vi "Conversao Ms to Hora texto.vi"(1 "TRUE=HORA\nFALSE=GRAU":bool, 2 "PrecDEC":dbl caption="DEC arcsec" format="%.3g") -> (0 "Hora/Graus Texto Decimal":string)   [LabVIEW 2018]
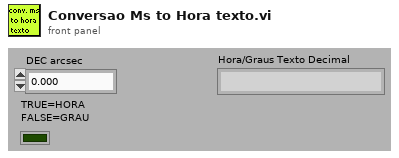
[diagram p1: front panel]
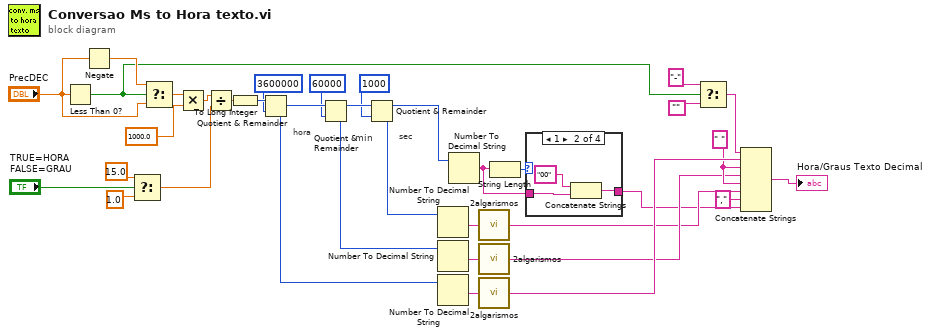
[diagram p0: block diagram]
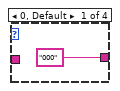
[diagram p2: hidden frame]
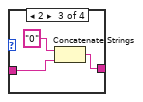
[diagram p3: hidden frame]
diagram:
  w22 = " " ("string")
  # "sec"
  # "min"
  # "hora"
  n1 = Less Than 0?(x="PrecDEC") -> (x < 0?=w9:bool)
  n2 = Negate(x="PrecDEC") -> (-x=w11:dbl)
  n3 = Select(t=15.0 ("y"), s="TRUE=HORA\nFALSE=GRAU", f=1.0 ("y")) -> (s? t:f=w1:dbl)
  n4 = Select(t=w11, s=w9, f="PrecDEC") -> (s? t:f=w13:dbl)
  n5 = Multiply(x=w13, y=1000.0) -> (x*y=w6:dbl)
  n6 = Divide(x=w6, y=w1) -> (x/y=w5:dbl)
  n7 = To Long Integer(number=w5) -> (32bit integer=w35:i32)
  n8 = Quotient & Remainder(x=w35, y=3600000) -> (x-y*floor(x/y)=w33:i32, floor(x/y)=w29:i32)
  n9 = Quotient & Remainder(x=w33, y=60000) -> (x-y*floor(x/y)=w31:i32, floor(x/y)=w25:i32)
  n10 = Quotient & Remainder(x=w31, y=1000) -> (x-y*floor(x/y)=w18:i32, floor(x/y)=w24:i32)
  n11 = Number To Decimal String(number=w24) -> (decimal integer string=w26:string)  [unwired: 1 in]
  n12 = Number To Decimal String(number=w25) -> (decimal integer string=w27:string)  [unwired: 1 in]
  n13 = Number To Decimal String(number=w29) -> (decimal integer string=w28:string)  [unwired: 1 in]
  n14 = Number To Decimal String(number=w18) -> (decimal integer string=w16:string)  [unwired: 1 in]
  n15 = call "2algarismos.vi"("entrada"=w26) -> ("saida"=w20:string)
  n16 = call "2algarismos.vi"("entrada"=w27) -> ("saida"=w21:string)
  n17 = call "2algarismos.vi"("entrada"=w28) -> ("saida"=w23:string)
  n18 = String Length(string=w16) -> (length=w17:i32)
  n19 = case shown="1" w17 {
    tunnel: w16 -> [_ w40 w42 w44]
    tunnel: ["000" ("string") w38 w41 w44] -> w15
    frame 0, Default {
    }
    frame 1 {
      n20 = Concatenate Strings("00" ("string"), w40) -> (w38:string)
    }
    frame 2 {
      n21 = Concatenate Strings("0" ("string"), w42) -> (w41:string)
    }
    frame 3 {
    }
  }
  n22 = Select(t="-" ("string"), s=w9, f="") -> (s? t:f=w7:string)
  n23 = Concatenate Strings(w7, w23, w22, w21, w22, w20, "," ("string"), w15) -> (→"Hora/Graus Texto Decimal":string)
